vi "gjson_RecursiveParser.vi"(11 "Json string":string) -> (2 "result string 2":string, 3 "String":string)   [LabVIEW 2015, in "Json2Labv.lvlib"]
uses:
  Json2Labv.lvlib
  <vilib>/regexp/Match Regular Expression.xnode
panel:
  out "match substring":string
  out "before substring":string
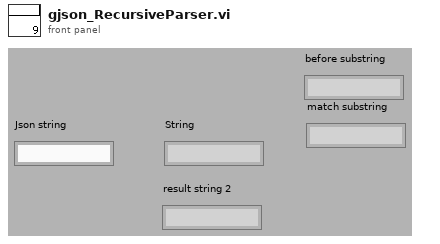
[diagram p1: front panel]
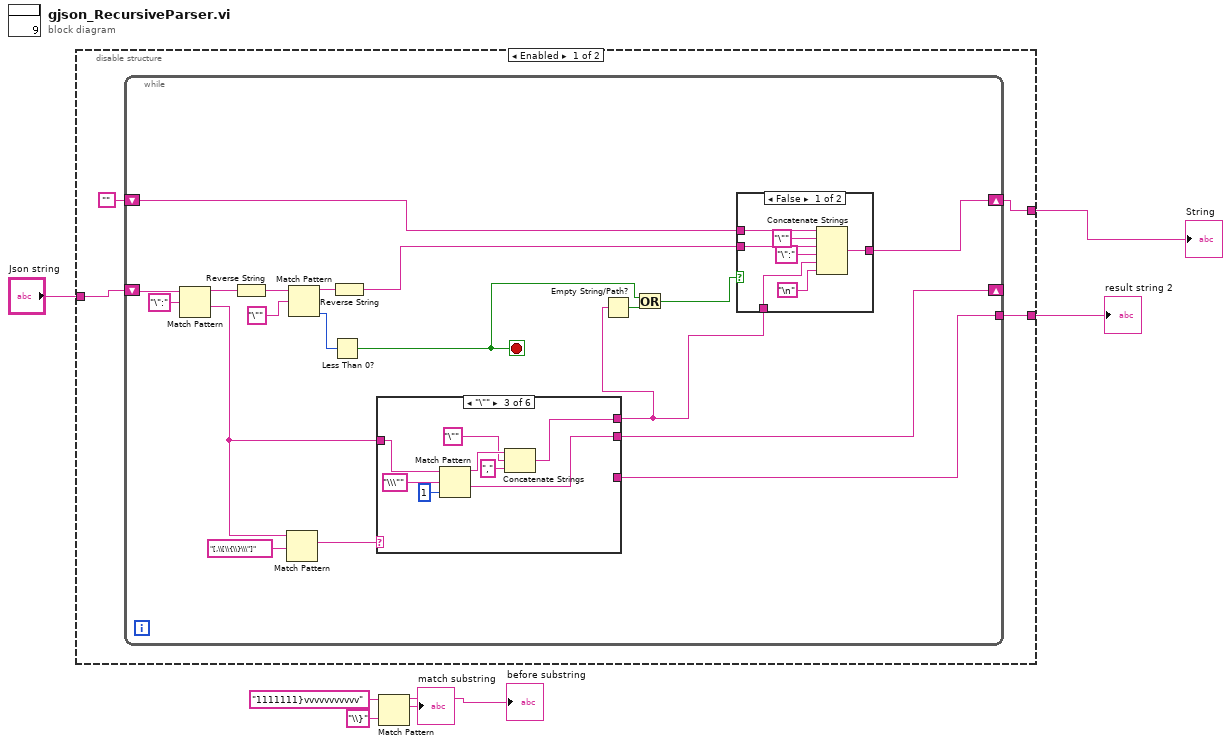
[diagram p0: block diagram]
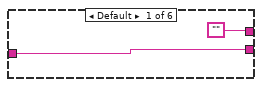
[diagram p3: hidden frame]
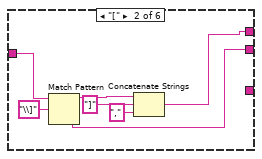
[diagram p4: hidden frame]
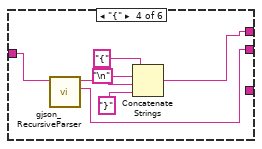
[diagram p5: hidden frame]
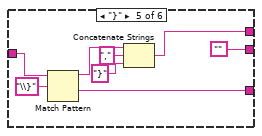
[diagram p6: hidden frame]
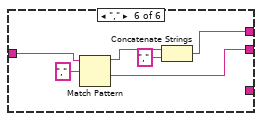
[diagram p7: hidden frame]
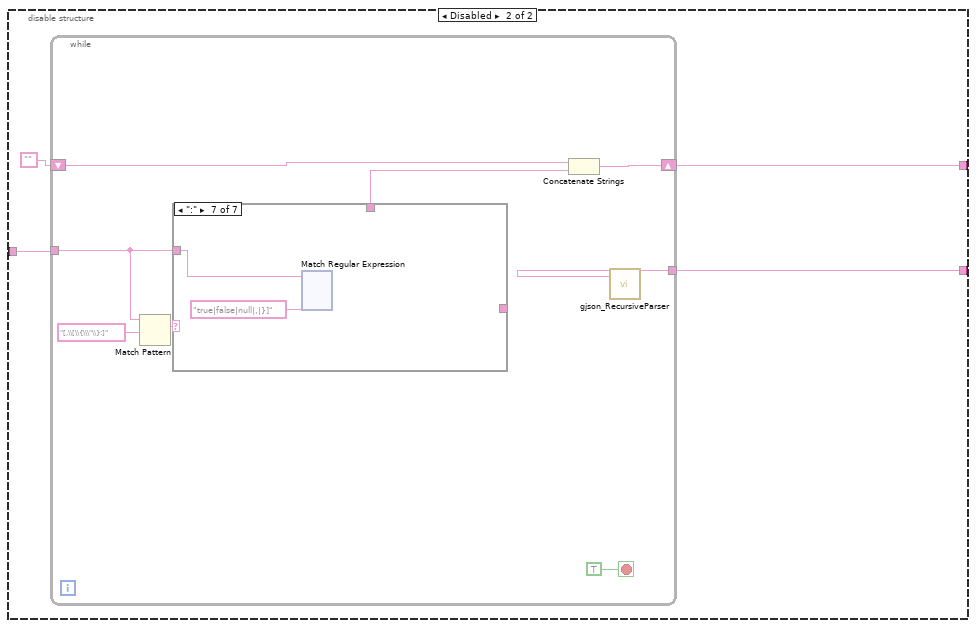
[diagram p8: hidden frame]
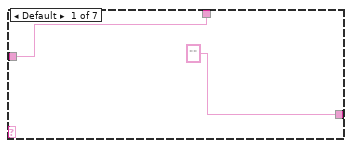
[diagram p9: hidden frame]
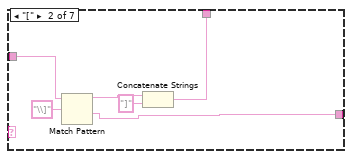
[diagram p10: hidden frame]
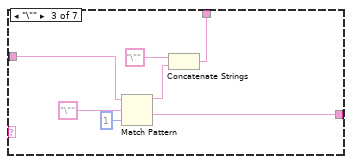
[diagram p11: hidden frame]
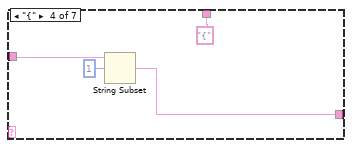
[diagram p12: hidden frame]
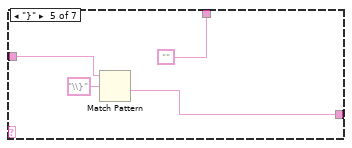
[diagram p13: hidden frame]
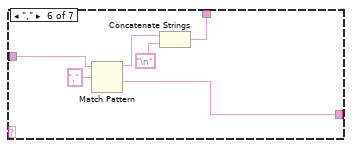
[diagram p14: hidden frame]
diagram:
  n1 = disable-structure shown="Enabled" {
    disable-tunnel: "Json string" -> [w11 w80]
    disable-tunnel: [w9 w78] -> w6
    disable-tunnel: [w8 w77] -> w5
    frame Enabled {
      n2 = while {
        shift-right: [w22] -> _
        shift-left: w11 -> [w30]
        shift-right: [w27] -> w9
        shift-left: "" -> [w18]
        tunnel: [w17] -> w8
        stop <- w14 stop-if-true
        n3 = Match Pattern(string=w30, regular expression="\":") -> (before substring=w26:string, after substring=w20:string)  [unwired: 1 in, 2 out]
        n4 = Reverse String(1:w26) -> (0:w25:string)
        n5 = Match Pattern(string=w20, regular expression="[,\\[\\{\\}\\\"]") -> (match substring=w19:string)  [unwired: 1 in, 3 out]
        n6 = Match Pattern(string=w25, regular expression="\"") -> (before substring=w24:string, offset past match=w23:i32)  [unwired: 1 in, 2 out]
        n7 = Less Than 0?(x=w23) -> (x < 0?=w14:bool)
        n8 = Reverse String(1:w24) -> (0:w16:string)
        n9 = case shown="\"\\\"\"" w19 {
          tunnel: w20 -> [w40 w47 w55 w60 w70 w76]
          tunnel: [w40 w44 w52 w59 "" w74] -> w22
          tunnel: [_ _ _ _ w68 _] -> w17
          tunnel: ["" w41 w48 w56 w65 w71] -> w12
          frame Default {
          }
          frame "[" {
            n10 = Match Pattern(string=w47, regular expression="\\]") -> (before substring=w45:string, after substring=w44:string)  [unwired: 1 in, 2 out]
            n11 = Concatenate Strings(w45, "]" ("string"), "," ("string")) -> (w41:string)
          }
          frame "\"" {
            n12 = Match Pattern(string=w55, regular expression="\\\"", offset (0)=1) -> (before substring=w53:string, after substring=w52:string)  [unwired: 2 out]
            n13 = Concatenate Strings(w53, "\"" ("string"), "," ("string")) -> (w48:string)
          }
          frame "{" {
            n14 = call "gjson_RecursiveParser.vi"("Json string"=w60) -> ("result string 2"=w59:string, "String"=w62:string)  [unwired: 9 in]
            n15 = Concatenate Strings("{" ("string"), "\n", w62, "}" ("string")) -> (w56:string)
          }
          frame "}" {
            n16 = Match Pattern(string=w70, regular expression="\\}") -> (before substring=w66:string, after substring=w68:string)  [unwired: 1 in, 2 out]
            n17 = Concatenate Strings(w66, "," ("string"), "}" ("string")) -> (w65:string)
          }
          frame "," {
            n18 = Match Pattern(string=w76, regular expression=",") -> (before substring=w73:string, after substring=w74:string)  [unwired: 1 in, 2 out]
            n19 = Concatenate Strings(w73, "," ("string")) -> (w71:string)
          }
        }
        n20 = Empty String/Path?(string/path=w12) -> (empty?=w13:bool)
        n21 = Or(x=w14, y=w13) -> (x .or. y?=w15:bool)
        n22 = case shown="False" w15 {
          tunnel: [w37 w38] -> w27
          tunnel: w12 -> [w34 _]
          tunnel: w18 -> [w33 w38]
          tunnel: w16 -> [w31 _]
          frame False {
            n23 = Concatenate Strings(w33, "\"" ("string"), w31, "\":" ("string"), w34, "\n") -> (w37:string)
          }
          frame True {
          }
        }
      }
    }
    frame Disabled {
      n24 = while {
        shift-right: [w84] -> w78
        shift-left: "" -> [w83]
        tunnel: w80 -> [w86]
        tunnel: [w81] -> w77
        stop <- TRUE stop-if-true
        n25 = Match Pattern(string=w86, regular expression="[,\\[\\{\\\"\\}:]") -> (match substring=w87:string)  [unwired: 1 in, 3 out]
        n26 = case shown="\":\"" w87 {
          tunnel: w86 -> [w89 w93 w101 w107 w110 w116 w118]
          tunnel: ["" ("result string") w91 w100 w105 w109 w115 _] -> _
          tunnel: [w89 w92 w99 "{" "" w113 _] -> w82
          frame Default {
          }
          frame "[" {
            n27 = Match Pattern(string=w93, regular expression="\\]") -> (before substring=w95:string, after substring=w91:string)  [unwired: 1 in, 2 out]
            n28 = Concatenate Strings(w95, "]" ("string")) -> (w92:string)
          }
          frame "\"" {
            n29 = Match Pattern(string=w101, regular expression="\"", offset (0)=1) -> (before substring=w98:string, after substring=w100:string)  [unwired: 2 out]
            n30 = Concatenate Strings("\"" ("string"), w98) -> (w99:string)
          }
          frame "{" {
            n31 = String Subset(string=w107, offset (0)=1) -> (substring=w105:string)  [unwired: 1 in]
          }
          frame "}" {
            n32 = Match Pattern(string=w110, regular expression="\\}") -> (after substring=w109:string)  [unwired: 1 in, 3 out]
          }
          frame "," {
            n33 = Match Pattern(string=w116, regular expression=",") -> (before substring=w114:string, after substring=w115:string)  [unwired: 1 in, 2 out]
            n34 = Concatenate Strings(w114, "\n") -> (w113:string)
          }
          frame ":" {
            n35 = xnode "Match Regular Expression"("input string"=w118, "regular expression"="true|false|null|,|}]") -> ()  [unwired: 4 in, 5 out]
          }
        }
        n36 = Concatenate Strings(w83, w82) -> (w84:string)
        n37 = call "gjson_RecursiveParser.vi"() -> ("String"=w81:string)  [unwired: 1 in, 1 out]
      }
    }
  }
  "String" <- w6
  "result string 2" <- w5
  n38 = Match Pattern(string="1111111}vvvvvvvvvvv", regular expression="\\}") -> (before substring=→"before substring":string, match substring=→"match substring":string)  [unwired: 1 in, 2 out]
